vi "Configure Impedance.vi"(8 "error in (no error)":errorcluster, 10 "Impedance (1: 100kOhm)":i32(ring)=1 items=["50Ohm", "100kOhm"], 11 "VISA resource name":refnum<visa-resource-name>) -> (0 "error out":errorcluster, 3 "VISA resource name out":refnum<visa-resource-name>)   [LabVIEW 2014, in "Agilent U2000 Series.lvlib"]
doc: "Configures the impedance of the trigger input port.\n\nNote:\nThis VI supports model U2020 X-Series and U2040 X-Series only."
uses:
  Agilent U2000 Series.lvlib
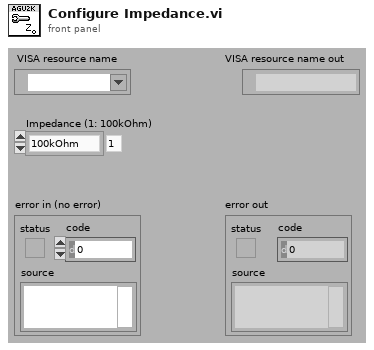
[diagram p1: front panel]
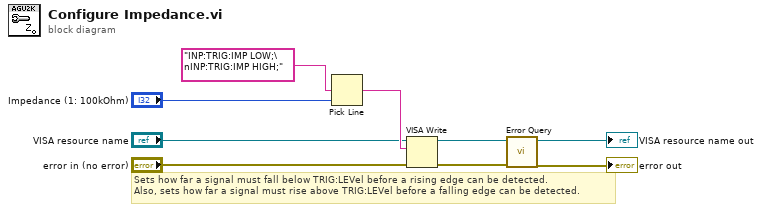
[diagram p0: block diagram]
diagram:
  # "Sets how far a signal must fall below TRIG:LEVel before a rising edge can be detected.\nAlso, sets how far a signal must rise above TRIG:LEVel before a falling edge can be detected."
  n1 = Pick Line(multi-line string="INP:TRIG:IMP LOW;\nINP:TRIG:IMP HIGH;", line index="Impedance (1: 100kOhm)") -> (output string=w7:string)  [unwired: 1 out]
  n2 = VISA Write(VISA resource name="VISA resource name", write buffer=w7, error in (no error)="error in (no error)") -> (VISA resource name out=w4:refnum<visa-resource-name>, error out=w3:errorcluster)  [unwired: 1 out]
  n3 = call "Error Query.vi"("error in (no error)"=w3, "VISA resource name"=w4) -> ("error out"=→"error out":errorcluster, "VISA resource name out"=→"VISA resource name out":refnum<visa-resource-name>)  [unwired: 8 out]
